vi "ReversedEngineering ViCachMemory.vi"(0 "ViRef":refnum<vi>, 1 "ViRef-Array":refnum<vi>[](array[refnum]), 2 "RemoveAllCachedViRefs(False)":bool, 3 "error in (no error)":errorcluster) -> (17 "error out":errorcluster)   [LabVIEW 2020]
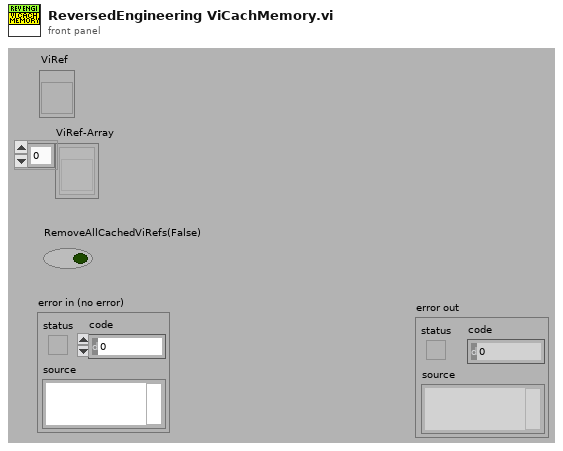
[diagram p1: front panel]
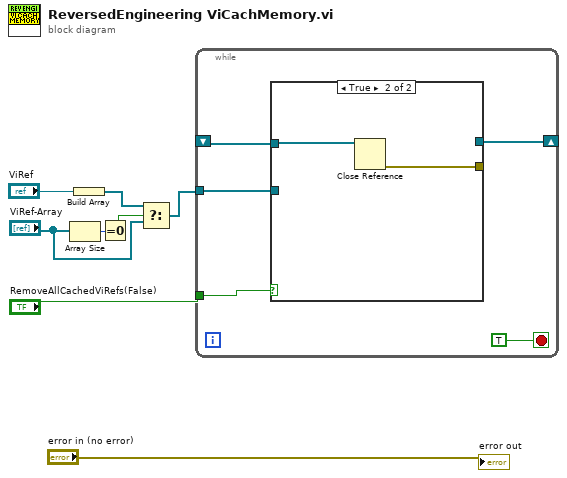
[diagram p0: block diagram]
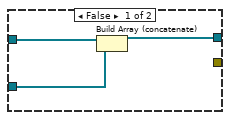
[diagram p2: hidden frame]
diagram:
  n1 = Array Size(array="ViRef-Array") -> (size(s)=w6:i32)
  n2 = Build Array("ViRef") -> (w1:refnum<vi>[])
  n3 = Equal To 0?(x=w6) -> (x = 0?=w5:bool)
  n4 = Select(t=w1, s=w5, f="ViRef-Array") -> (s? t:f=w2:refnum<vi>[])
  n5 = while {
    shift-right: [w11] -> _
    shift-left: _ -> [w13]
    tunnel: w2 -> [w12]
    tunnel: "RemoveAllCachedViRefs(False)" -> [w9]
    stop <- TRUE stop-if-true
    n6 = case shown="True" w9 {
      tunnel: w13 -> [w16 w18]
      tunnel: w12 -> [w15 _]
      tunnel: [w14 _] -> w11
      tunnel: [_ w17] -> _
      frame False {
        n7 = Build Array (concatenate)(w16, w15) -> (w14:refnum<vi>[])
      }
      frame True {
        n8 = Close Reference(reference=w18) -> (error out=w17:errorcluster)  [unwired: 1 in]
      }
    }
  }
  "error out" <- "error in (no error)"
